vi "test1-TestModuleStatusVI.vi"(8 "error in (no error)":errorcluster, 11 "TestCase in":refnum<class "testcase-CSMManagementAPI.lvclass">) -> (0 "error out":errorcluster, 3 "TestCase out":refnum<class "testcase-CSMManagementAPI.lvclass">)   [LabVIEW 2017, in "testcase-CSMManagementAPI.lvclass"]
uses:
  testcase-CSMManagementAPI.lvclass
  src/user.lib/_NEVSTOP/Communicable State Machine(CSM)/_Support/Typedef/_CSM_List Module Scope.ctl
  src/user.lib/_NEVSTOP/Communicable State Machine(CSM)/_Support/Typedef/_CSM_MODE.ctl
  src/user.lib/_NEVSTOP/Communicable State Machine(CSM)/AdvanceAPI/CSM - Revert Arguments-Safe String.vi
  src/user.lib/_NEVSTOP/Communicable State Machine(CSM)/AdvanceAPI/CSM - Make String Arguments Safe.vi
  src/user.lib/_NEVSTOP/Communicable State Machine(CSM)/AdvanceAPI/CSM - Break Down Multiple States String.vi
  src/user.lib/_NEVSTOP/Communicable State Machine(CSM)/AdvanceAPI/CSM - Compact Multiple States.vi
  src/user.lib/_NEVSTOP/Communicable State Machine(CSM)/AdvanceAPI/CSM - Keywords.vi
  src/user.lib/_NEVSTOP/Communicable State Machine(CSM)/_Shared/Trim Single-line Text.vi
  <vilib>/addons/_JKI Toolkits/VI Tester/TestCase.llb/TestCase.lvclass
  src/user.lib/_NEVSTOP/Communicable State Machine(CSM)/Communicable State Machine.lvlib
  C:/Program Files (x86)/National Instruments/LabVIEW 2017/vi.lib/addons/_JKI Toolkits/VI Tester/TestCase.llb/TestCase.lvclass
panel:
  out "State History":string
  out "error out 2":errorcluster
  out "LoopCount":i32
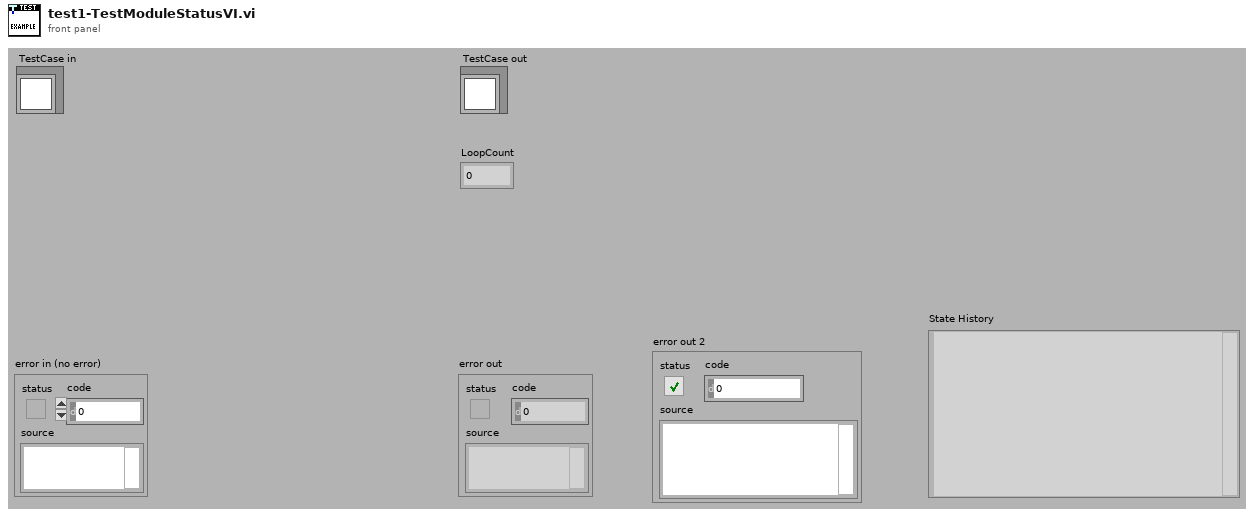
[diagram p1: front panel]
types:
  T1 = typedef "Communicable State Machine.lvlib/_CSM_MODE.ctl" = enum16{"Not Exist", "Stand Alone", "CSM", "Worker", "Worker Agent", "Chain Node", "Chain"}
  T2 = cluster{"CSM Name (Dup)":string, "Mode":T1, "#Nodes":i32}[]
  T3 = typedef "Communicable State Machine.lvlib/_CSM_List Module Scope.ctl" = enum16{"Normal", "System Only", "All"}
  T4 = enum32{"Invalid", "Standard", "Closed", "Hidden", "Minimized", "Maximized"}
  T5 = enum32{"invalid app kind", "Development System", "Run Time System", "Student Edition", "Embedded LabVIEW", "Evaluation", "Custom"}
  T6 = typedef "Communicable State Machine.lvlib/_CSM_Response Source Message.ctl" = cluster{"‘State":string, "’Arguments":string, "’Error":errorcluster}
  T7 = cluster{"Current VI Reference":refnum<vi>, "Close Panel on Exit?":bool}
  T8 = cluster{"Core":cluster{"Current VI Reference":refnum<vi>, "Close Panel on Exit?":bool}, "Your Boolean data":bool, "Your string data":string, "Module Status":cluster{"CSM Name (Dup)":string, "Mode":T1, "#Nodes":i32}}
  T9 = cluster{"CSM Name (Dup)":string, "Mode":T1, "#Nodes":i32}
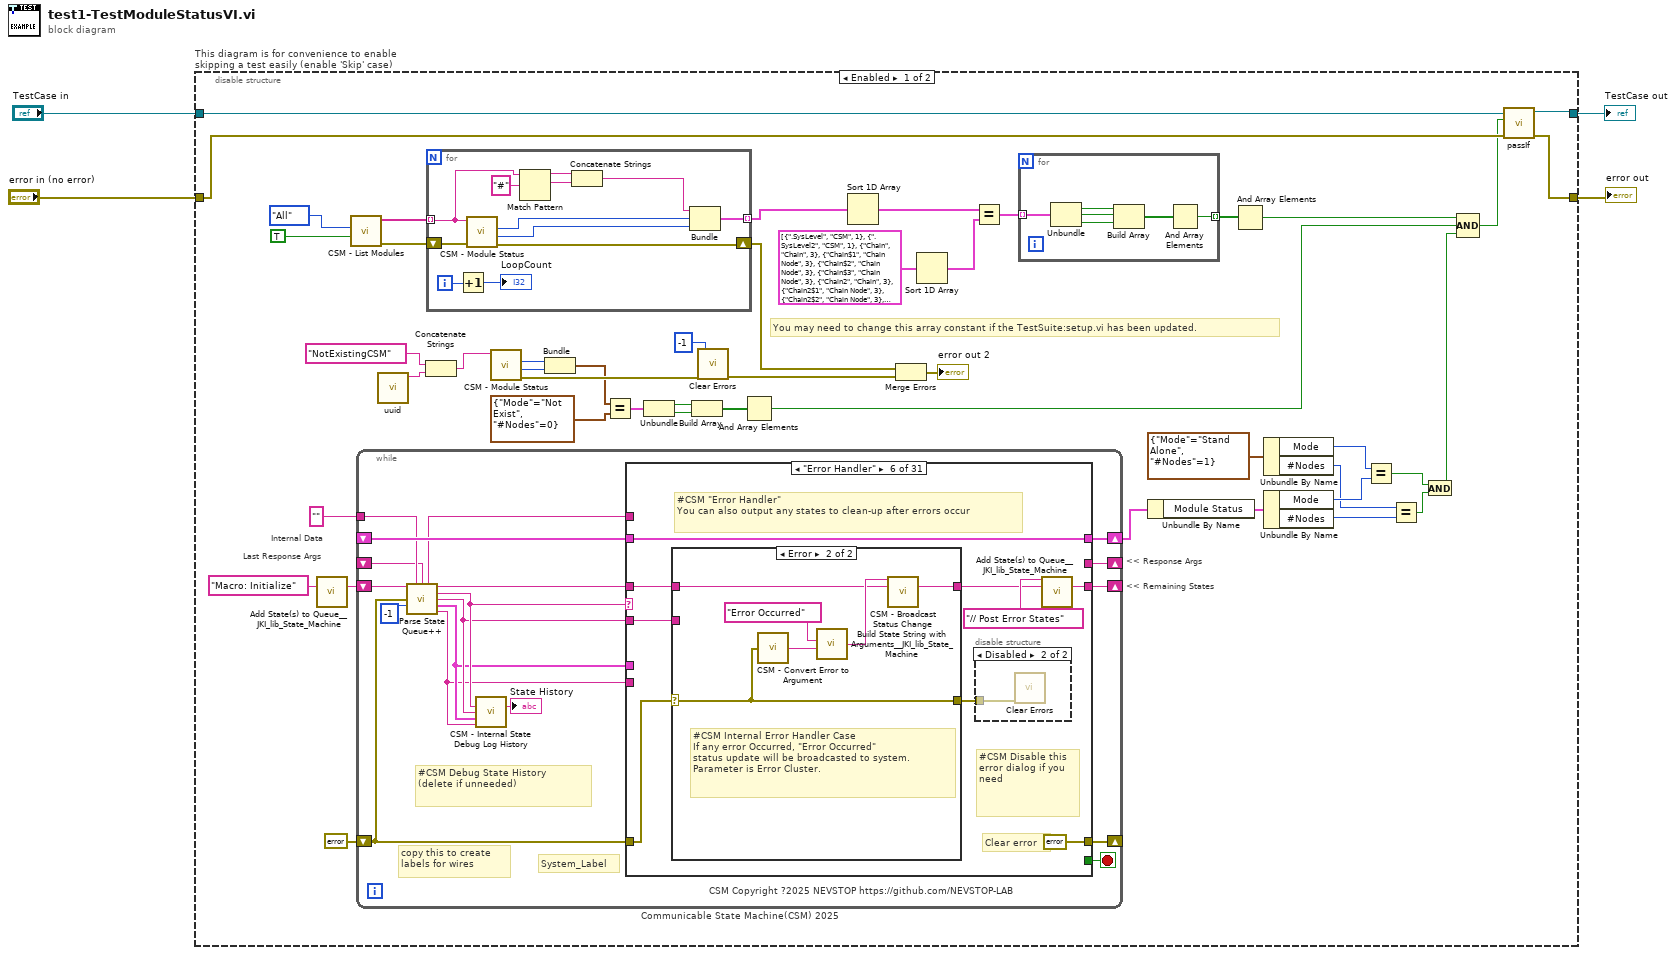
[diagram p0: block diagram]
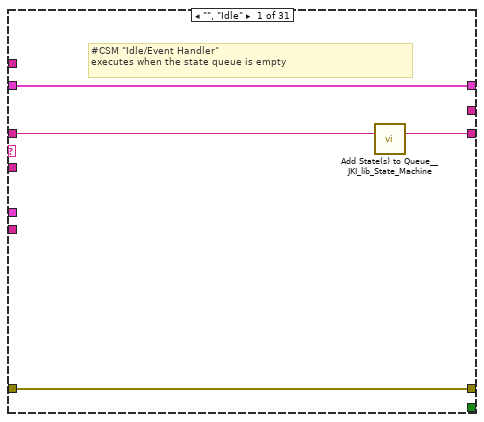
[diagram p2: hidden frame]
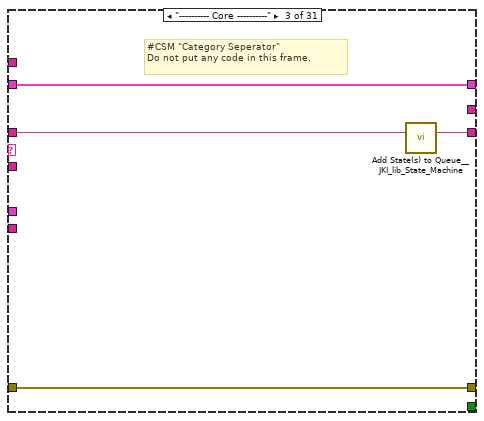
[diagram p4: hidden frame]
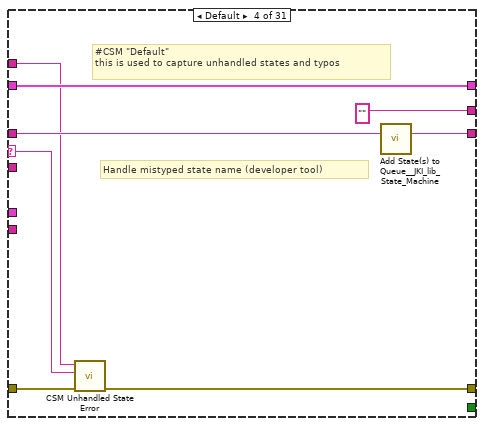
[diagram p5: hidden frame]
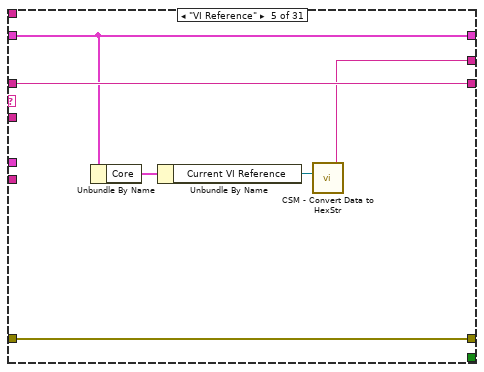
[diagram p6: hidden frame]
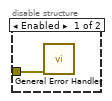
[diagram p7: hidden frame]
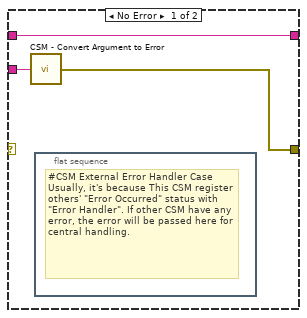
[diagram p8: hidden frame]
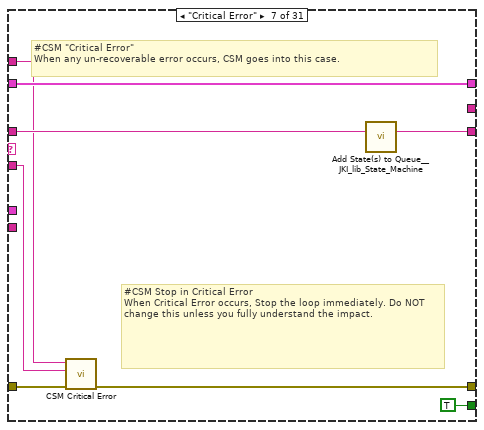
[diagram p9: hidden frame]
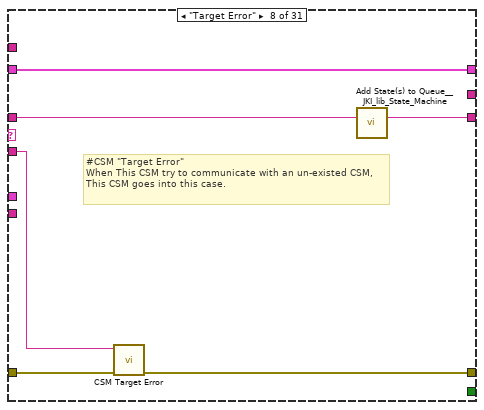
[diagram p10: hidden frame]
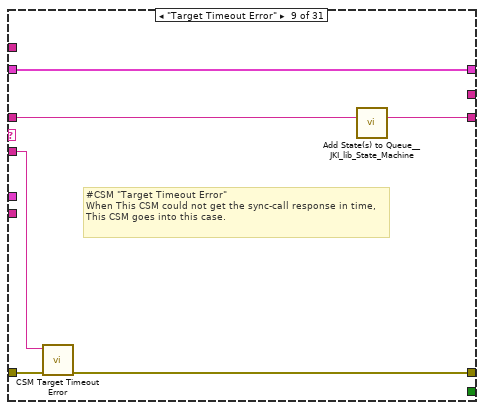
[diagram p11: hidden frame]
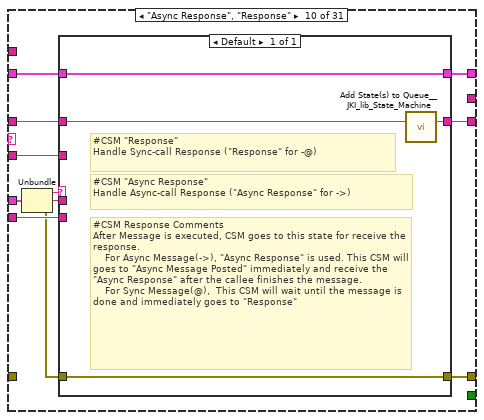
[diagram p12: hidden frame]
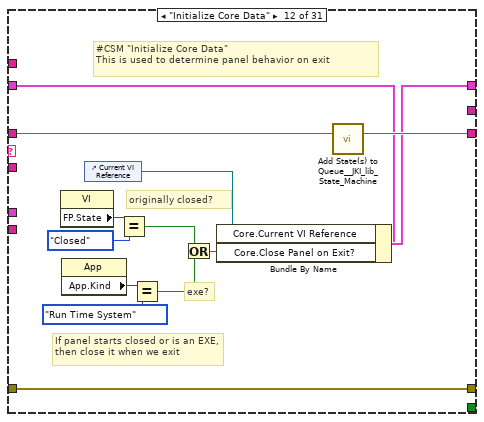
[diagram p14: hidden frame]
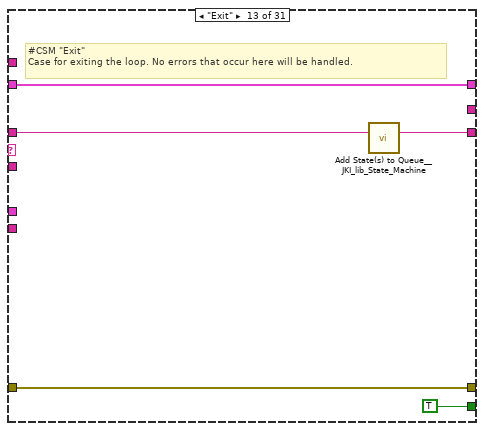
[diagram p15: hidden frame]
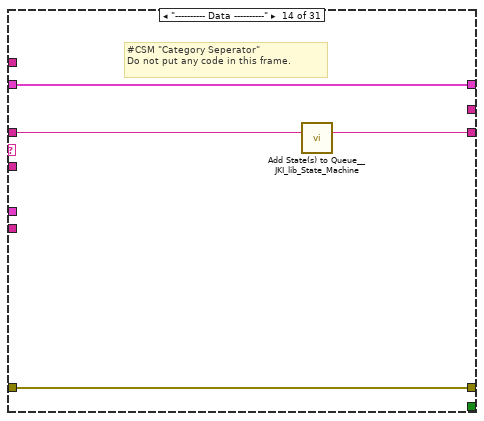
[diagram p16: hidden frame]
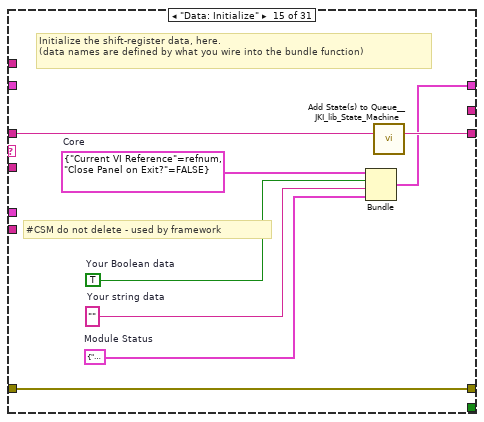
[diagram p17: hidden frame]
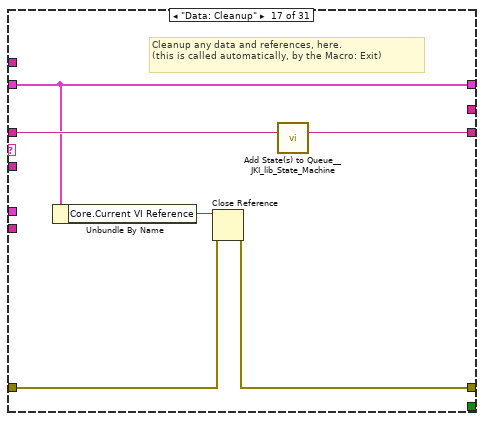
[diagram p19: hidden frame]
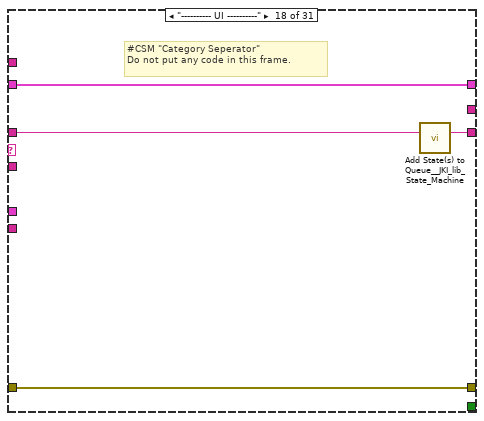
[diagram p20: hidden frame]
diagram:
  n1 = disable-structure "This diagram is for convenience to enable skipping a test easily (enable 'Skip' case)" shown="Enabled" {
    disable-tunnel: "TestCase in" -> [w47 w361]
    disable-tunnel: [w46 w359] -> w1
    disable-tunnel: [w44 w360] -> w3
    disable-tunnel: "error in (no error)" -> [w45 w358]
    frame Enabled {
      # "You may need to change this array constant if the TestSuite:setup.vi has been updated."
      # "Last Response Args"
      # "Internal Data"
      # "<< Response Args"
      # "<< Remaining States"
      n2 = call <vilib>:"Add State(s) to Queue__JKI_lib_State_Machine.vi"("State(s) in (\"\")"="Macro: Initialize" ("Init State(\"Macro: Initialize\")")) -> ("States Out"=w39:string)  [unwired: 14 in]
      n3 = call "CSM - List Modules.vi"("With Nodes? (F)"=TRUE, "Scope (Normal)"=_CSM_List_Module_Scope."All") -> ("error out"=w49:errorcluster, "Module Names"=w48:string[])  [unwired: 8 in]
      n4 = while "Communicable State Machine(CSM) 2025" {
        shift-right: [w70] -> w38
        shift-left: _ -> [w69]
        shift-right: [w73] -> _
        shift-left: errorcluster {"status"=FALSE, "code"=0, "source"=""} ("error out") -> [w68]
        shift-right: [w72] -> _
        shift-left: w39 -> [w74]
        tunnel: "" ("Name (\"\" to Use UUID)") -> [w66]
        shift-right: [w67] -> _
        shift-left: _ -> [w60]
        stop <- w71 stop-if-true
        # "#CSM Debug State History\n(delete if unneeded)"
        # "copy this to create labels for wires"
        # "System_Label"
        # "CSM Copyright ?2025 NEVSTOP https://github.com/NEVSTOP-LAB"
        n5 = call "Parse State Queue++.vi"("State Queue"=w74, "Name (\"\" to Use UUID)"=w66, "Response Arguments"=w60, "Previous Error"=w68, "Dequeue (1 ms)"=-1 ("Timeout")) -> ("Name Used"=w61:string, "Remaining States"=w75:string, "Current State"=w65:string, "Arguments"=w64:string, "Additional Information"=w63:T6, "Source CSM"=w62:string)  [unwired: 5 in]
        n6 = call "CSM - Internal State Debug Log History.vi"("State"=w65, "Arguments (\"\")"=w64, ">> Response Source Message >>"=w63, "Source (\"\")"=w62) -> ("Debug Log"=→"State History":string)  [unwired: 11 in]
        n7 = case shown="\"Error Handler\"" w65 {
          selector: w65 -> [_ _ _ w89 _ _ _ _ _ _ _ _ _ _ _ _ _ _ _ _ _ _ _ _ _ _ _ _ _ _ _]
          tunnel: w75 -> [w76 w81 w86 w93 w99 w105 w126 w132 w138 w146 w157 w171 w176 w180 w188 w190 w197 w201 w205 w211 w226 w295 w300 w307 w309 w313 w318 w325 w329 w333 w345]
          tunnel: w64 -> [_ _ _ _ _ w104 w122 w131 w136 w145 _ _ _ _ _ _ _ _ _ w206 w220 _ _ _ _ _ w316 _ _ _ _]
          tunnel: w69 -> [w77 w80 w83 w91 w98 w108 w127 w133 w139 w148 w156 w164 w174 w177 _ w189 w192 w198 w203 w209 w222 w292 w297 w304 w308 w312 w317 w322 w326 w330 w338]
          tunnel: [w78 w82 w84 w87 w100 errorcluster {"status"=FALSE, "code"=0, "source"=""} ("error out") w123 w129 w135 w151 w158 w168 w173 w178 w185 w191 w193 w199 w202 w207 w223 w293 w298 w305 w310 w314 w319 w323 w327 w331 w335] -> w73
          tunnel: w68 -> [w78 w82 w84 w94 w100 w106 w128 w130 w137 _ w158 w168 w173 w178 w185 w191 w194 w199 w202 w208 w224 w293 w298 w305 w310 w314 w319 w323 w327 w331 w343]
          tunnel: [w79 w81 w85 w92 w99 w101 w125 w134 w140 w147 w157 w170 w175 w179 w187 w190 w196 w200 w204 w210 w225 w294 w299 w306 w309 w313 w318 w324 w328 w332 w344] -> w72
          tunnel: [_ _ _ _ _ _ TRUE _ _ _ _ _ TRUE _ _ _ _ _ _ _ _ _ _ _ _ _ _ _ _ _ _] -> w71
          tunnel: [w77 w80 w83 w91 w98 w108 w127 w133 w139 w149 w156 w169 w174 w177 w186 w189 w192 w198 w203 w209 w222 w292 w297 w304 w308 w312 w317 w322 w326 w330 w337] -> w70
          tunnel: w62 -> [_ _ _ _ _ _ _ _ _ w143 _ _ _ _ _ _ _ _ _ _ _ _ _ _ _ _ _ _ _ _ _]
          tunnel: w63 -> [_ _ _ _ _ _ _ _ _ w150 _ _ _ _ _ _ _ _ _ _ _ _ _ _ _ _ _ _ _ _ _]
          tunnel: [_ _ _ "" w95 _ _ _ _ _ _ _ _ _ _ _ _ _ _ _ _ _ _ _ _ "API1 Response" w315 _ _ _ _] -> w67
          tunnel: w61 -> [_ _ _ w88 _ _ w121 _ _ _ _ _ _ _ _ _ _ _ _ _ _ _ _ _ _ _ _ _ _ _ w342]
          frame "", "Idle" {
            # "#CSM \"Idle/Event Handler\"\nexecutes when the state queue is empty"
            n8 = call <vilib>:"Add State(s) to Queue__JKI_lib_State_Machine.vi"("State(s) in (\"\")"=w76) -> ("States Out"=w79:string)  [unwired: 14 in]
          }
          frame "CSM Documentation" {
            # "#CSM README FIRST\n\nCommunicable State Machine(CSM) is a LabVIEW application framework that builds upon JKI State Machine(JKISM). It follows the pattern of JKISM and extends the keywords to describe message communication between modules, including concepts such as Sync-Message, Async-Message, Subscription/Unsubscription of status - essential elements for creating reusable code modules. For more information, please visit the CSM wiki: https://nevstop-lab.github.io/CSM-Wiki/\n\nFor instructions on JKI State Machine, visit: http://jki.net/state-machine/\nFor information about CSM, visit: https://github.com/NEVSTOP-LAB"
            # "#CSM \"Documentation\"\nCase for holding CSM Documenation"
          }
          frame "---------- Core ----------" {
            # "#CSM \"Category Seperator\"\nDo not put any code in this frame."
            n9 = call <vilib>:"Add State(s) to Queue__JKI_lib_State_Machine.vi"("State(s) in (\"\")"=w86) -> ("States Out"=w85:string)  [unwired: 14 in]
          }
          frame Default {
            # "#CSM \"Default\"\nthis is used to capture unhandled states and typos"
            # "Handle mistyped state name (developer tool)"
            n10 = call "CSM Unhandled State Error.vi"("error in (no error)"=w94, "Undefined State"=w89, "CSM Name"=w88) -> ("error out"=w87:errorcluster)  [unwired: 8 in]
            n11 = call <vilib>:"Add State(s) to Queue__JKI_lib_State_Machine.vi"("State(s) in (\"\")"=w93) -> ("States Out"=w92:string)  [unwired: 14 in]
          }
          frame "VI Reference" {
            n12 = Unbundle By Name(w98) -> ("Core"=w97:T7)
            n13 = Unbundle By Name(w97) -> ("Current VI Reference"=w96:refnum<vi>)
            n14 = call "CSM - Convert Data to HexStr.vi"("Variant"=w96) -> ("HEX String (0-9,A-F)"=w95:string)  [unwired: 8 in]
          }
          frame "Error Handler" {
            # "#CSM Disable this error dialog if you need"
            # "#CSM \"Error Handler\"\nYou can also output any states to clean-up after errors occur"
            # "Clear error"
            n15 = case shown="Error" w106 {
              selector: w106 -> [_ w115]
              tunnel: [w114 w117] -> w102
              tunnel: w105 -> [w114 w116]
              tunnel: w104 -> [w113 _]
              tunnel: [w112 w115] -> w107
              frame No Error {
                n16 = call "CSM - Convert Argument to Error.vi"("Argument"=w113) -> ("Error"=w112:errorcluster)  [unwired: 4 in]
                n17 = flat-sequence {
                  frame #0 {
                    # "#CSM External Error Handler Case\nUsually, it's because This CSM register others' \"Error Occurred\" status with \"Error Handler\". If other CSM have any error, the error will be passed here for central handling."
                  }
                }
              }
              frame Error {
                # "#CSM Internal Error Handler Case \nIf any error Occurred, \"Error Occurred\" \nstatus update will be broadcasted to system.\nParameter is Error Cluster."
                n18 = call "CSM - Convert Error to Argument.vi"("Error"=w115) -> ("Argument"=w119:string)  [unwired: 4 in]
                n19 = call <vilib>:"Build State String with Arguments__JKI_lib_State_Machine.vi"("Arguments (\"\")"=w119, "State"="Error Occurred" ("Status with Arguments")) -> ("State with Arguments"=w118:string)  [unwired: 4 in]
                n20 = call "CSM - Broadcast Status Change.vi"("Status With Arguments"=w118, "State Queue"=w116) -> ("Remaining States"=w117:string)  [unwired: 13 in]
              }
            }
            n21 = disable-structure shown="Disabled" {
              disable-tunnel: w107 -> [w110 w111]
              frame Enabled {
                n22 = call <vilib>:"General Error Handler.vi"("error in (no error)"=w110) -> ()  [unwired: 10 in, 5 out]
              }
              frame Disabled {
                n23 = call <vilib>:"Clear Errors.vi"("error in (no error)"=w111) -> ()  [unwired: 5 in, 2 out]
              }
            }
            n24 = call <vilib>:"Add State(s) to Queue__JKI_lib_State_Machine.vi"("State(s) in Front (\"\")"="// Post Error States", "State(s) in (\"\")"=w102) -> ("States Out"=w101:string)  [unwired: 13 in]
          }
          frame "Critical Error" {
            # "#CSM Stop in Critical Error\nWhen Critical Error occurs, Stop the loop immediately. Do NOT change this unless you fully understand the impact."
            # "#CSM \"Critical Error\"\nWhen any un-recoverable error occurs, CSM goes into this case."
            n25 = call "CSM Critical Error.vi"("error in (no error)"=w128, "Arugments (As Reason)"=w122, "CSM Name"=w121) -> ("error out"=w123:errorcluster)  [unwired: 8 in]
            n26 = call <vilib>:"Add State(s) to Queue__JKI_lib_State_Machine.vi"("State(s) in (\"\")"=w126) -> ("States Out"=w125:string)  [unwired: 14 in]
          }
          frame "Target Error" {
            # "#CSM \"Target Error\"\nWhen This CSM try to communicate with an un-existed CSM, This CSM goes into this case."
            n27 = call "CSM Target Error.vi"("error in (no error)"=w130, "Arguments (As CSM Name)"=w131) -> ("error out"=w129:errorcluster)  [unwired: 9 in]
            n28 = call <vilib>:"Add State(s) to Queue__JKI_lib_State_Machine.vi"("State(s) in (\"\")"=w132) -> ("States Out"=w134:string)  [unwired: 14 in]
          }
          frame "Target Timeout Error" {
            # "#CSM \"Target Timeout Error\"\nWhen This CSM could not get the sync-call response in time, This CSM goes into this case."
            n29 = call "CSM Target Timeout Error.vi"("error in (no error)"=w137, "Arguments (As CSM Name)"=w136) -> ("error out"=w135:errorcluster)  [unwired: 9 in]
            n30 = call <vilib>:"Add State(s) to Queue__JKI_lib_State_Machine.vi"("State(s) in (\"\")"=w138) -> ("States Out"=w140:string)  [unwired: 14 in]
          }
          frame "Async Response", "Response" {
            n31 = Unbundle(w150) -> ("‘State"=w144:string, "’Arguments"=w142:string, "’Error"=w141:errorcluster)
            n32 = case shown="Default" w144 {
              tunnel: [w155] -> w151
              tunnel: w141 -> [w155]
              tunnel: [w154] -> w149
              tunnel: w148 -> [w154]
              tunnel: [w152] -> w147
              tunnel: w146 -> [w153]
              tunnel: w145 -> [_]
              tunnel: w143 -> [_]
              tunnel: w142 -> [_]
              frame Default {
                # "#CSM Response Comments\nAfter Message is executed, CSM goes to this state for receive the response.\n    For Async Message(->), \"Async Response\" is used. This CSM will goes to \"Async Message Posted\" immediately and receive the \"Async Response\" after the callee finishes the message.\n    For Sync Message(@),  This CSM will wait until the message is done and immediately goes to \"Response\""
                # "#CSM \"Async Response\"\nHandle Async-call Response (\"Async Response\" for ->)"
                # "#CSM \"Response\"\nHandle Sync-call Response (\"Response\" for -@)"
                n33 = call <vilib>:"Add State(s) to Queue__JKI_lib_State_Machine.vi"("State(s) in (\"\")"=w153) -> ("States Out"=w152:string)  [unwired: 14 in]
              }
            }
          }
          frame "Async Message Posted" {
            # "#CSM \"Async Message Posted\"\nAfter Async Message is posted (-> or ->| ), CSM goes to this state for post-action.\nYou can use Argument - State to tell which Async Message is called."
          }
          frame "Initialize Core Data" {
            # "#CSM \"Initialize Core Data\"\nThis is used to determine panel behavior on exit"
            # "originally closed?"
            # "exe?"
            # "If panel starts closed or is an EXE, then close it when we exit"
            n34 = property class="VI"() -> ("FP.State"=w161:T4)  [unwired: 2 in, 2 out]
            n35 = property class="App"() -> ("App.Kind"=w167:T5)  [unwired: 2 in, 2 out]
            n36 = control-ref of="Current VI Reference"() -> (w162:refnum<vi>)
            n37 = Equal?(x=w161, y=T4."Closed" ("Front Panel Window:State")) -> (x = y?=w159:bool)
            n38 = Equal?(x=w167, y=T5."Run Time System" ("Application:Kind")) -> (x = y?=w165:bool)
            n39 = Or(x=w159, y=w165) -> (x .or. y?=w163:bool)
            n40 = Bundle By Name(cluster=w164, "Core.Current VI Reference"=w162, "Core.Close Panel on Exit?"=w163) -> (w169:T8)
            n41 = call <vilib>:"Add State(s) to Queue__JKI_lib_State_Machine.vi"("State(s) in (\"\")"=w171) -> ("States Out"=w170:string)  [unwired: 14 in]
          }
          frame "Exit" {
            # "#CSM \"Exit\"\nCase for exiting the loop. No errors that occur here will be handled."
            n42 = call <vilib>:"Add State(s) to Queue__JKI_lib_State_Machine.vi"("State(s) in (\"\")"=w176) -> ("States Out"=w175:string)  [unwired: 14 in]
          }
          frame "---------- Data ----------" {
            # "#CSM \"Category Seperator\"\nDo not put any code in this frame."
            n43 = call <vilib>:"Add State(s) to Queue__JKI_lib_State_Machine.vi"("State(s) in (\"\")"=w180) -> ("States Out"=w179:string)  [unwired: 14 in]
          }
          frame "Data: Initialize" {
            w181 = T9 {"CSM Name (Dup)"="", "Mode"=enum."Not Exist", "#Nodes"=0}  # Module Status
            w182 = T7 {"Current VI Reference"=refnum, "Close Panel on Exit?"=FALSE}  # Core
            w184 = TRUE  # Your Boolean data
            w183 = ""  # Your string data
            # "#CSM do not delete - used by framework"
            # "Initialize the shift-register data, here.\n(data names are defined by what you wire into the bundle function)"
            n44 = Bundle("Core"=w182, "Your Boolean data"=w184, "Your string data"=w183, "Module Status"=w181) -> (w186:T8)  [unwired: 1 in]
            n45 = call <vilib>:"Add State(s) to Queue__JKI_lib_State_Machine.vi"("State(s) in (\"\")"=w188) -> ("States Out"=w187:string)  [unwired: 14 in]
          }
          frame "Data: Update Indicators" {
          }
          frame "Data: Cleanup" {
            # "Cleanup any data and references, here.\n(this is called automatically, by the Macro: Exit)"
            n46 = Unbundle By Name(w192) -> ("Core.Current VI Reference"=w195:refnum<vi>)
            n47 = Close Reference(reference=w195, error in (no error)=w194) -> (error out=w193:errorcluster)
            n48 = call <vilib>:"Add State(s) to Queue__JKI_lib_State_Machine.vi"("State(s) in (\"\")"=w197) -> ("States Out"=w196:string)  [unwired: 14 in]
          }
          frame "---------- UI ----------" {
            # "#CSM \"Category Seperator\"\nDo not put any code in this frame."
            n49 = call <vilib>:"Add State(s) to Queue__JKI_lib_State_Machine.vi"("State(s) in (\"\")"=w201) -> ("States Out"=w200:string)  [unwired: 14 in]
          }
          frame "UI: Initialize" {
            # "#CSM \"UI: Initialize\"\nInitialize the User Interface, here.\n(this is called automatically, by the Macro: Init)"
            n50 = call <vilib>:"Add State(s) to Queue__JKI_lib_State_Machine.vi"("State(s) in (\"\")"=w205) -> ("States Out"=w204:string)  [unwired: 14 in]
          }
          frame "UI: Cursor Set" {
            # "#CSM \"UI: Cursor Set\"\nSet and Unset Cursor Busy.\n(Usage: \"UI: Cursor Set >> Busy|Idle\")"
            # "Argument"
            n51 = disable-structure shown="TARGET_TYPE!=Windows" {
              disable-tunnel: w208 -> [w214 w219]
              disable-tunnel: [w213 w219] -> w207
              disable-tunnel: w206 -> [w212 _]
              frame condition #0 (active) {
                n52 = case shown="\"Idle\", Default" w212 {
                  tunnel: w214 -> [w216 w218]
                  tunnel: [w215 w217] -> w213
                  frame "Idle", Default {
                    n53 = call <vilib>:"Unset Busy.vi"("error in (no error)"=w216) -> ("error out"=w215:errorcluster)  [unwired: 10 in]
                  }
                  frame "Busy" {
                    n54 = call <vilib>:"Set Busy.vi"("error in (no error)"=w218) -> ("error out"=w217:errorcluster)  [unwired: 9 in, 1 out]
                  }
                }
              }
              frame condition #1 {
              }
            }
            n55 = call <vilib>:"Add State(s) to Queue__JKI_lib_State_Machine.vi"("State(s) in (\"\")"=w211) -> ("States Out"=w210:string)  [unwired: 14 in]
          }
          frame "UI: Front Panel State" {
            # "#CSM \"UI: Front Panel State\"\nSet Front Panel Open or Closed\n(Usage: \"UI: Front Panel State >> Open|Close\")"
            # "Argument"
            n56 = Unbundle By Name(w222) -> ("Core.Current VI Reference"=w221:refnum<vi>)
            n57 = call <vilib>:"Add State(s) to Queue__JKI_lib_State_Machine.vi"("State(s) in (\"\")"=w226) -> ("States Out"=w225:string)  [unwired: 14 in]
            n58 = case shown="\"Close\", \"Closed\"" w220 {
              tunnel: w224 -> [w232 w247 w258 w271 w284]
              tunnel: [w234 w248 w260 w273 w286] -> w223
              tunnel: w221 -> [w233 w245 w259 w272 w285]
              frame "Open", "Standard", Default {
                w227 = T4."Standard" ("State")
                n59 = property class="VI"(reference=w233, error in=w232) -> (reference out=w230:refnum<vi>, error out=w231:errorcluster, "FP.State"=w229:T4)
                n60 = Not Equal?(x=w229, y=w227) -> (x != y?=w228:bool)
                n61 = case shown="True" w228 {
                  tunnel: [w238 w240] -> w234
                  tunnel: w231 -> [w237 w240]
                  tunnel: w230 -> [w236 _]
                  tunnel: w227 -> [w235 _]
                  frame True {
                    n62 = invoke class="VI" method="FP.Open"(reference=w236, error in=w237, "Activate"=TRUE, "State"=w235) -> (error out=w238:errorcluster)  [unwired: 1 in, 4 out]
                  }
                  frame False {
                  }
                }
              }
              frame "Close", "Closed" {
                n63 = property class="VI"(reference=w245, error in=w247) -> (reference out=w244:refnum<vi>, error out=w246:errorcluster, "FP.State"=w242:T4)
                n64 = Not Equal?(x=w242, y=T4."Closed" ("Front Panel Window:State")) -> (x != y?=w241:bool)
                n65 = case shown="False" w241 {
                  tunnel: [w249 w252] -> w248
                  tunnel: w246 -> [w249 w251]
                  tunnel: w244 -> [_ w250]
                  frame False {
                  }
                  frame True {
                    n66 = invoke class="VI" method="FP.Close"(reference=w250, error in=w251) -> (error out=w252:errorcluster)  [unwired: 1 in, 2 out]
                  }
                }
              }
              frame "Hidden", "Hide" {
                w253 = T4."Hidden" ("State")
                n67 = property class="VI"(reference=w259, error in=w258) -> (reference out=w256:refnum<vi>, error out=w257:errorcluster, "FP.State"=w255:T4)
                n68 = Not Equal?(x=w255, y=w253) -> (x != y?=w254:bool)
                n69 = case shown="True" w254 {
                  tunnel: [w264 w265] -> w260
                  tunnel: w257 -> [w263 w265]
                  tunnel: w256 -> [w262 _]
                  tunnel: w253 -> [w261 _]
                  frame True {
                    n70 = invoke class="VI" method="FP.Open"(reference=w262, error in=w263, "State"=w261) -> (error out=w264:errorcluster)  [unwired: 2 in, 4 out]
                  }
                  frame False {
                  }
                }
              }
              frame "Minimize", "Minimized" {
                w266 = T4."Minimized" ("State")
                n71 = property class="VI"(reference=w272, error in=w271) -> (reference out=w269:refnum<vi>, error out=w270:errorcluster, "FP.State"=w268:T4)
                n72 = Not Equal?(x=w268, y=w266) -> (x != y?=w267:bool)
                n73 = case shown="True" w267 {
                  tunnel: [w277 w278] -> w273
                  tunnel: w270 -> [w276 w278]
                  tunnel: w269 -> [w275 _]
                  tunnel: w266 -> [w274 _]
                  frame True {
                    n74 = invoke class="VI" method="FP.Open"(reference=w275, error in=w276, "State"=w274) -> (error out=w277:errorcluster)  [unwired: 2 in, 4 out]
                  }
                  frame False {
                  }
                }
              }
              frame "Maximize", "Maximized" {
                w279 = T4."Maximized" ("State")
                n75 = property class="VI"(reference=w285, error in=w284) -> (reference out=w282:refnum<vi>, error out=w283:errorcluster, "FP.State"=w281:T4)
                n76 = Not Equal?(x=w281, y=w279) -> (x != y?=w280:bool)
                n77 = case shown="True" w280 {
                  tunnel: [w290 w291] -> w286
                  tunnel: w283 -> [w289 w291]
                  tunnel: w282 -> [w288 _]
                  tunnel: w279 -> [w287 _]
                  frame True {
                    n78 = invoke class="VI" method="FP.Open"(reference=w288, error in=w289, "State"=w287) -> (error out=w290:errorcluster)  [unwired: 2 in, 4 out]
                  }
                  frame False {
                  }
                }
              }
            }
          }
          frame "---------- Macro ----------" {
            # "#CSM \"Category Seperator\"\nDo not put any code in this frame."
            n79 = call <vilib>:"Add State(s) to Queue__JKI_lib_State_Machine.vi"("State(s) in (\"\")"=w295) -> ("States Out"=w294:string)  [unwired: 14 in]
          }
          frame "Macro: Initialize" {
            # "#CSM \"Macro: Initialize\"\nInitialization Macro (This is called once, when the VI starts)"
            n80 = call <vilib>:"Add State(s) to Queue__JKI_lib_State_Machine.vi"("State(s) in Front (\"\")"="Data: Initialize\nInitialize Core Data\nData: Update Indicators\nAction: Check Module Status\nMacro: Exit", "State(s) in (\"\")"=w300) -> ("States Out"=w299:string)  [unwired: 13 in]
          }
          frame "Macro: Exit" {
            # "#CSM \"Macro: Exit\"\nExit Macro (This is called once, when the VI exits)"
            n81 = call <vilib>:"Add State(s) to Queue__JKI_lib_State_Machine.vi"("State(s) in Front (\"\")"="//Exit Sub-Modules ", "State(s) at Back (\"\")"="Data: Cleanup\nExit") -> ("States Out"=w302:string)  [unwired: 13 in]
            n82 = call <vilib>:"Add State(s) to Queue__JKI_lib_State_Machine.vi"("State(s) in Front (\"\")"=w302, "State(s) in (\"\")"=w307) -> ("States Out"=w306:string)  [unwired: 13 in]
          }
          frame "---------- API ----------" {
            # "#CSM \"Category Seperator\"\nDo not put any code in this frame."
          }
          frame "API: API1" {
            # "#CSM API Example\nCopy/Rename this case for your own API"
            # "#CSM Response\nConnect this to return the response of your API"
            # "#CSM >> Msg/Rep's CSM >>\nIf you need to tell who triggered this state , use this string. If it's this case itself, this string is \"\"."
            # "#CSM >> Arguments >>\nDeal with the parameter if any"
          }
          frame "API: API2" {
            # "#CSM API Example\nCopy/Rename this case for your own API"
            # "unpack Hex String  to Variant\nif complex parameter is needed."
            n83 = call "CSM - Convert HexStr to Data.vi"("HEX String"=w316) -> ()  [unwired: 7 in, 2 out]
            n84 = disable-structure shown="Disabled" {
              disable-tunnel: [w320 "API2 Response"] -> w315
              frame Disabled {
                # "pack variant to hexstr \nif complex response is needed."
                # "complex Response"
                n85 = call "CSM - Convert Data to HexStr.vi"() -> ("HEX String (0-9,A-F)"=w320:string)  [unwired: 9 in]
              }
              frame Enabled {
              }
            }
          }
          frame "---------- Action ----------" {
            # "#CSM \"Category Seperator\"\nDo not put any code in this frame."
            n86 = call <vilib>:"Add State(s) to Queue__JKI_lib_State_Machine.vi"("State(s) in (\"\")"=w325) -> ("States Out"=w324:string)  [unwired: 14 in]
          }
          frame "Action: action1" {
            # "#CSM \"Internal State\"\nThis category is used for holding internal states"
            n87 = call <vilib>:"Add State(s) to Queue__JKI_lib_State_Machine.vi"("State(s) in (\"\")"=w329) -> ("States Out"=w328:string)  [unwired: 14 in]
          }
          frame "Action: action2" {
            # "#CSM \"Internal State\"\nThis category is used for holding internal states"
            n88 = call <vilib>:"Add State(s) to Queue__JKI_lib_State_Machine.vi"("State(s) in (\"\")"=w333) -> ("States Out"=w332:string)  [unwired: 14 in]
          }
          frame "Action: Check Module Status" {
            n89 = call "CSM - Module Status.vi"("CSM Name"=w342) -> ("error out"=w334:errorcluster, "#Nodes"=w339:i32, "Mode"=w340:T1, "CSM Name (Dup)"=w341:string)  [unwired: 6 in, 1 out]
            n90 = Bundle("CSM Name (Dup)"=w341, "Mode"=w340, "#Nodes"=w339) -> (w336:T9)  [unwired: 1 in]
            n91 = Bundle By Name(cluster=w338, "Module Status"=w336) -> (w337:T8)
            n92 = Merge Errors(w343, w334) -> (w335:errorcluster)
            n93 = call <vilib>:"Add State(s) to Queue__JKI_lib_State_Machine.vi"("State(s) in (\"\")"=w345) -> ("States Out"=w344:string)  [unwired: 14 in]
          }
        }
      }
      n94 = call "uuid.vi"() -> ("UUID"=w30:string)  [unwired: 11 in]
      n95 = Concatenate Strings("NotExistingCSM" ("CSM Name"), w30) -> (w29:string)
      n96 = for {
        tunnel: w48 -> [w349] mode=indexing
        shift-right: [w356] -> w43
        shift-left: w49 -> [w357]
        tunnel: [w351] -> w28 mode=indexing
        i -> [w355]
        n97 = Increment(x=w355) -> (x+1=→"LoopCount":i32)
        n98 = call "CSM - Module Status.vi"("Error In"=w357, "CSM Name"=w349) -> ("error out"=w356:errorcluster, "#Nodes"=w352:i32, "Mode"=w353:T1)  [unwired: 5 in, 2 out]
        n99 = Match Pattern(string=w349, regular expression="#") -> (before substring=w348:string, match substring=w347:string)  [unwired: 1 in, 2 out]
        n100 = Concatenate Strings(w348, w347) -> (w346:string)
        n101 = Bundle(w346, "Mode"=w353, "#Nodes"=w352) -> (w351:cluster{string, "Mode":T1, "#Nodes":i32})  [unwired: 1 in]
      }
      n102 = call "CSM - Module Status.vi"("CSM Name"=w29) -> ("error out"=w34:errorcluster, "#Nodes"=w36:i32, "Mode"=w37:T1)  [unwired: 6 in, 2 out]
      n103 = Bundle("Mode"=w37, "#Nodes"=w36) -> (w21:cluster{"Mode":T1, "#Nodes":i32})  [unwired: 1 in]
      n104 = Equal?(x=w21, y=cluster{"Mode":T1, "#Nodes":i32} {"Mode"=enum."Not Exist", "#Nodes"=0} ("Module Status")) -> (x = y?=w19:cluster{"Mode":bool, "#Nodes":bool})
      n105 = Unbundle(w19) -> ("Mode"=w18:bool, "#Nodes"=w17:bool)
      n106 = Build Array(w18, w17) -> (w16:bool[])
      n107 = call <vilib>:"Clear Errors.vi"("error in (no error)"=w34, "specific error code to clear (0: all)"=-1) -> ("error out"=w33:errorcluster)  [unwired: 4 in, 1 out]
      n108 = And Array Elements(Boolean array=w16) -> (logical AND=w15:bool)
      n109 = Sort 1D Array(array=w28) -> (sorted array=w26:cluster{string, "Mode":T1, "#Nodes":i32}[])
      n110 = Merge Errors(w43, w33) -> (→"error out 2":errorcluster)
      n111 = Sort 1D Array(array=T2 [{"CSM Name (Dup)"=".SysLevel", "Mode"=enum."CSM", "#Nodes"=1}, {"CSM Name (Dup)"=".SysLevel2", "Mode"=enum."CSM", "#Nodes"=1}, {"CSM Name (Dup)"="Chain", "Mode"=enum."Chain", "#Nodes"=3}, {"CSM Name (Dup)"="Chain$1", "Mode"=enum."Chain Node", "#Nodes"=3}, {"CSM Name (Dup)"="Chain$2", "Mode"=enum."Chain Node", "#Nodes"=3}, {"CSM Name (Dup)"="Chain$3", "Mode"=enum."Chain Node", "#Nodes"=3}, {"CSM Name (Dup)"="Chain2", "Mode"=enum."Chain", "#Nodes"=3}, {"CSM Name (Dup)"="Chain2$1", "Mode"=enum."Chain Node", "#Nodes"=3}, {"CSM Name (Dup)"="Chain2$2", "Mode"=enum."Chain Node", "#Nodes"=3}, {"CSM Name (Dup)"="Chain2$3", "Mode"=enum."Chain Node", "#Nodes"=3}, {"CSM Name (Dup)"="lvlibp", "Mode"=enum."CSM", "#Nodes"=1}, {"CSM Name (Dup)"="lvlibp2", "Mode"=enum."CSM", "#Nodes"=1}, {"CSM Name (Dup)"="Normal", "Mode"=enum."CSM", "#Nodes"=1}, {"CSM Name (Dup)"="Normal.SubModule", "Mode"=enum."CSM", "#Nodes"=1}, {"CSM Name (Dup)"="Normal.SubModule2", "Mode"=enum."CSM", "#Nodes"=1}, {"CSM Name (Dup)"="Normal2", "Mode"=enum."CSM", "#Nodes"=1}, {"CSM Name (Dup)"="worker", "Mode"=enum."Worker Agent", "#Nodes"=3}, {"CSM Name (Dup)"="worker#", "Mode"=enum."Worker", "#Nodes"=3}, {"CSM Name (Dup)"="worker#", "Mode"=enum."Worker", "#Nodes"=3}, {"CSM Name (Dup)"="worker#", "Mode"=enum."Worker", "#Nodes"=3}, {"CSM Name (Dup)"="worker2", "Mode"=enum."Worker Agent", "#Nodes"=3}, {"CSM Name (Dup)"="worker2#", "Mode"=enum."Worker", "#Nodes"=3}, {"CSM Name (Dup)"="worker2#", "Mode"=enum."Worker", "#Nodes"=3}, {"CSM Name (Dup)"="worker2#", "Mode"=enum."Worker", "#Nodes"=3}] ("Module Status Array 2")) -> (sorted array=w25:T2)
      n112 = Equal?(x=w26, y=w25) -> (x = y?=w24:cluster{bool, "Mode":bool, "#Nodes":bool}[])
      n113 = for {
        tunnel: w24 -> [w57] mode=indexing
        tunnel: [w52] -> w23 mode=indexing
        n114 = Unbundle(w57) -> (w56:bool, "Mode"=w55:bool, "#Nodes"=w54:bool)
        n115 = Build Array(w56, w55, w54) -> (w53:bool[])
        n116 = And Array Elements(Boolean array=w53) -> (logical AND=w52:bool)
      }
      n117 = Unbundle By Name(w38) -> ("Module Status"=w14:T9)
      n118 = And Array Elements(Boolean array=w23) -> (logical AND=w22:bool)
      n119 = Unbundle By Name(cluster{"Mode":T1, "#Nodes":i32} {"Mode"=enum."Stand Alone", "#Nodes"=1} ("Module Status")) -> ("Mode"=w12:T1, "#Nodes"=w10:i32)
      n120 = Unbundle By Name(w14) -> ("Mode"=w11:T1, "#Nodes"=w9:i32)
      n121 = Equal?(x=w12, y=w11) -> (x = y?=w7:bool)
      n122 = Equal?(x=w10, y=w9) -> (x = y?=w8:bool)
      n123 = And(x=w7, y=w8) -> (x .and. y?=w6:bool)
      n124 = Compound Arithmetic op=AND(w22, w15, w6) -> (w5:bool)
      n125 = call-dynamic "passIf.vi"("error in (no error)"=w45, "pass"=w5, "TestCase in"=w47) -> ("error out"=w44:errorcluster, "TestCase out"=w46:refnum<class "testcase-CSMManagementAPI.lvclass">)  [unwired: 7 in]
    }
    frame Disabled {
      # "skip test result while test is under development"
      n126 = call <vilib>:"skip.vi"("error in (no error)"=w358, "TestCase in"=w361) -> ("error out"=w360:errorcluster, "TestCase out"=w359:refnum<class "testcase-CSMManagementAPI.lvclass">)  [unwired: 8 in]
    }
  }
  "error out" <- w3
  "TestCase out" <- w1
